vi "LCR_Readout.vi"(8 "error in (no error)":errorcluster, 10 "Frequency in Hz":i32, 11 "HP4263B in":refnum<class "HP4263B.lvclass">) -> (0 "error out":errorcluster, 1 "Resistance in Ohm":dbl, 2 "Capacitance in pF":dbl, 3 "HP4263B out":refnum<class "HP4263B.lvclass">)   [LabVIEW 2013, in "HP4263B.lvclass"]
uses:
  HP4263B.lvclass
  InstrControl.lvclass
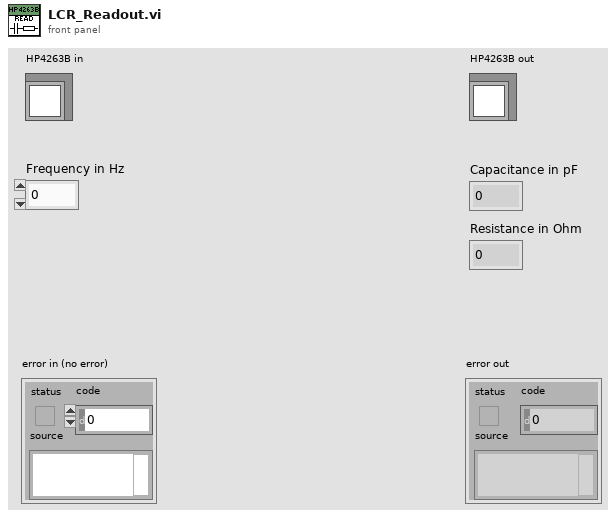
[diagram p1: front panel]
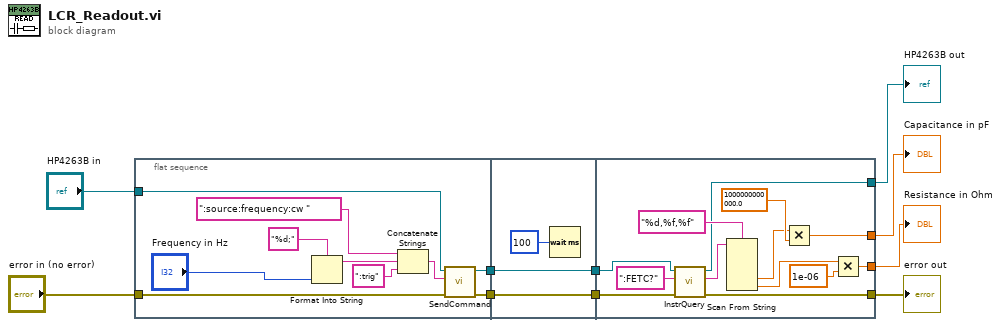
[diagram p0: block diagram]
diagram:
  n1 = flat-sequence {
    tunnel: "HP4263B in" -> [w14]
    tunnel: "error in (no error)" -> [w13]
    tunnel: [w12] -> w7
    tunnel: [w11] -> w5
    tunnel: [w22] -> w8
    tunnel: w7 -> [w22]
    tunnel: [w21] -> w6
    tunnel: w5 -> [w21]
    tunnel: w8 -> [w35]
    tunnel: w6 -> [w34]
    tunnel: [w27] -> w4
    tunnel: [w26] -> w3
    tunnel: [w25] -> w2
    tunnel: [w24] -> w1
    frame #0 {
      n2 = Format Into String(format string="%d;", "Frequency in Hz") -> (resulting string=w19:string)  [unwired: 2 in, 1 out]
      n3 = Concatenate Strings(":source:frequency:cw ", w19, ":trig") -> (w15:string)
      n4 = call "SendCommand.vi"("error in (no error)"=w13, "Command string"=w15, "InstControl in"=w14) -> ("error out"=w11:errorcluster, "InstControl out"=w12:refnum<class "HP4263B.lvclass">)  [unwired: 7 in]
    }
    frame #1 {
      n5 = Wait (ms)(milliseconds to wait=u32 100) -> ()  [unwired: 1 out]
    }
    frame #2 {
      n6 = call-dynamic "InstrQuery.vi"("error in (no error)"=w34, "Command string"=":FETC?", "InstControl in"=w35) -> ("error out"=w25:errorcluster, "Instrument response"=w28:string, "InstControl out"=w24:refnum<class "HP4263B.lvclass">)  [unwired: 6 in]
      n7 = Scan From String(format string="%d,%f,%f", input string=w28) -> (output 2=w30:dbl, output 3=w32:dbl)  [unwired: 6 in, 3 out]
      n8 = Multiply(x=w30, y=1000000000000.0) -> (x*y=w26:dbl)
      n9 = Multiply(x=w32, y=1e-06) -> (x*y=w27:dbl)
    }
  }
  "error out" <- w2
  "HP4263B out" <- w1
  "Capacitance in pF" <- w3
  "Resistance in Ohm" <- w4
